vi "ReportToFile.vi"(6 "Day":string, 8 "error in":errorcluster, 9 "Month":string, 10 "Report":string, 11 "dup path":path) -> (0 "error out":errorcluster)   [LabVIEW 2014]
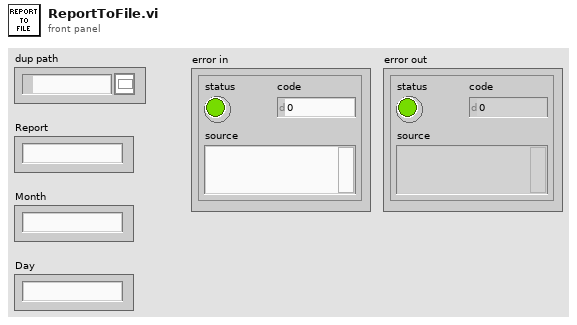
[diagram p1: front panel]
types:
  T1 = enum16{"open", "replace", "create", "open or create", "replace or create", "replace or create with confirmation"}
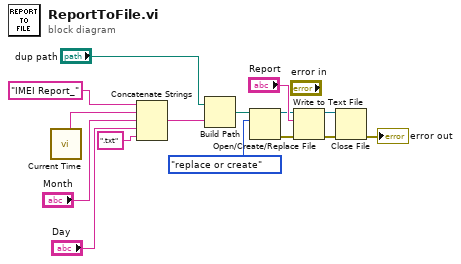
[diagram p0: block diagram]
diagram:
  n1 = call "Current Time.vi"() -> ("Year"=w9:string)  [unwired: 6 in, 5 out]
  n2 = Concatenate Strings("IMEI Report_", w9, "Month", "Day", ".txt") -> (w11:string)
  n3 = Build Path(base path="dup path", name or relative path=w11) -> (appended path=w7:path)
  n4 = Open/Create/Replace File(file path (use dialog)=w7, operation (0:open)=T1."replace or create") -> (refnum out=w2:refnum<file>, error out=w1:errorcluster)  [unwired: 4 in, 1 out]
  n5 = Write to Text File(file (use dialog)=w2, text="Report", error in=w1) -> (refnum out=w4:refnum<file>, error out=w3:errorcluster)  [unwired: 1 in, 1 out]
  n6 = Close File(refnum=w4, error in=w3) -> (error out=→"error out":errorcluster)  [unwired: 1 out]
